vi "Read maxEval.vi"(8 "error in (no error)":errorcluster, 11 "Objective in":refnum<class "Objective.lvclass">) -> (0 "error out":errorcluster, 2 "maxEval":dbl, 3 "Objective out":refnum<class "Objective.lvclass">)   [LabVIEW 2023, in "Objective.lvclass"]
uses:
  Objective.lvclass
  Objective.lvclass/Objective.ctl
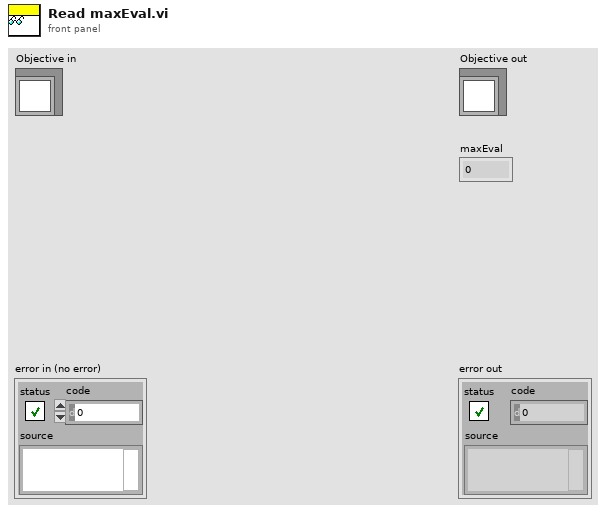
[diagram p1: front panel]
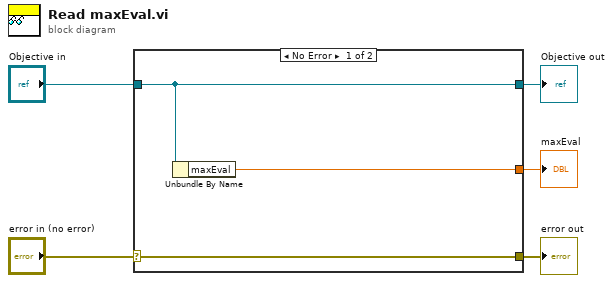
[diagram p0: block diagram]
diagram:
  n1 = case shown="No Error" "error in (no error)" {
    selector: "error in (no error)" -> [w8 w9]
    tunnel: [w8 w9] -> w4
    tunnel: [w7 w10] -> w2
    tunnel: "Objective in" -> [w7 w10]
    tunnel: [w6 _] -> w1
    frame No Error {
      n2 = Unbundle By Name(w7) -> ("maxEval"=w6:dbl)
    }
    frame Error {
    }
  }
  "error out" <- w4
  "Objective out" <- w2
  "maxEval" <- w1
